vi "CalMic-Initialize Hardware.vi"(0 "Device":string, 5 "Params":T1, 11 "error in (no error)":errorcluster) -> (4 "task out":refnum<k21>, 6 "RPcoX out":refnum<k7>, 8 "npts":i32, 15 "error out":errorcluster)   [LabVIEW 2020]
uses:
  CalMic-Params.ctl
  epl-vi-lib/PXI DAQ VIs/TDT VIs/TDT-Signal Bank Action.ctl
  3100642b-de6f-4996-8a80-97bce8963f67.vi
  <vilib>/Comparison/Equal/Equal Functor/Equal Functor.lvclass
  <vilib>/DAQmx/create/channels.llb/DAQmx Create Channel (AI-Voltage-Basic).vi
  <vilib>/DAQmx/configure/timing.llb/DAQmx Timing (Sample Clock).vi
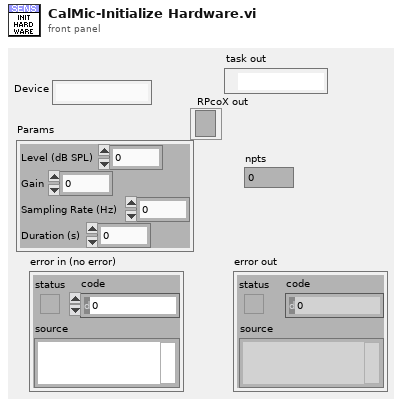
[diagram p1: front panel]
types:
  T1 = typedef "CalMic-Params.ctl" = cluster{"Level (dB SPL)":dbl, "Gain":dbl, "Sampling Rate (Hz)":dbl, "Duration (s)":dbl}
  T2 = typedef "TDT-Signal Bank Action.ctl" = enum16{"Init", "Write", "Read", "Rewrite", "Reset", "Recycle", "Ramp up", "Ramp down", "Zero"}
  T3 = typedef "TDT-Output source.ctl" = cluster{"Device":T4, "Num":i32}
  T4 = typedef "TDT-Device ID.ctl" = enum16{"None", "PA5", "RP2", "RL2", "RA16", "RV8", "RX5", "RX6", "RX7", "RX8", "RZ2", "RZ5", "RZ6"}
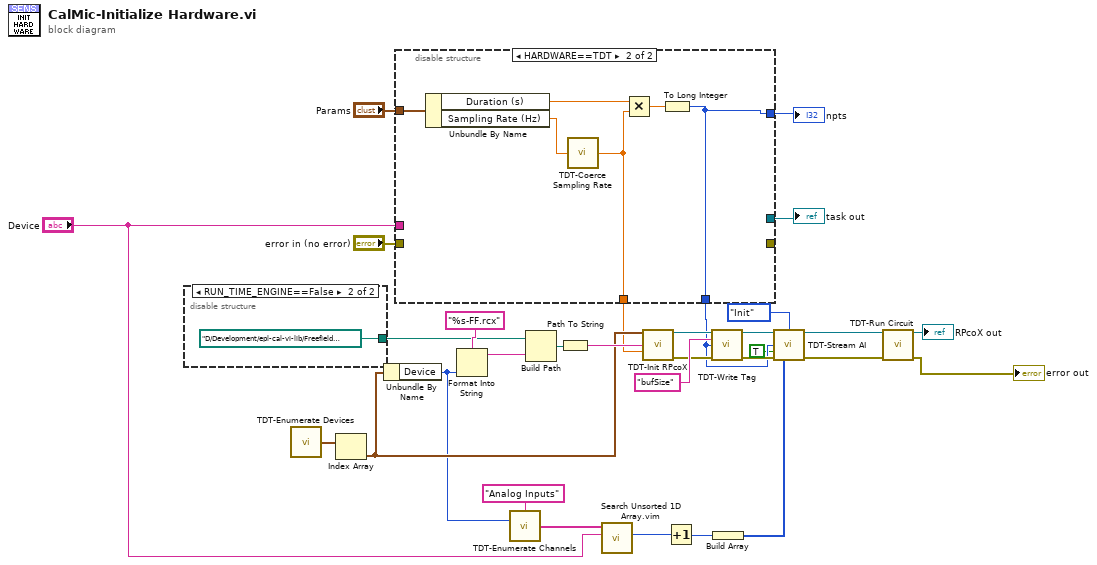
[diagram p0: block diagram]
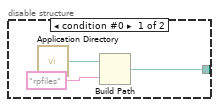
[diagram p2: hidden frame]
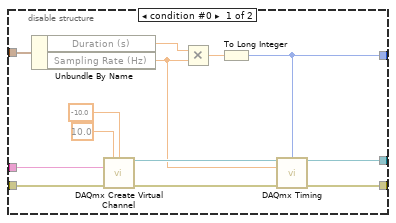
[diagram p3: hidden frame]
diagram:
  n1 = disable-structure shown="RUN_TIME_ENGINE==False" {
    disable-tunnel: [w33 path "D:/Development/epl-cal-vi-lib/Freefield Calibration VIs/rpfiles"] -> w23
    frame condition #0 {
      n2 = call <vilib>:"Application Directory.vi"() -> ("Application Directory"=w34:path)
      n3 = Build Path(base path=w34, name or relative path="rpfiles") -> (appended path=w33:path)
    }
    frame condition #1 (active) {
    }
  }
  n4 = call "TDT-Enumerate Devices.vi"() -> ("Devices"=w24:T3[])  [unwired: 14 in, 1 out]
  n5 = Index Array(array=w24) -> (element=w21:T3)  [unwired: 1 in]
  n6 = Unbundle By Name(w21) -> ("Device"=w15:T4)
  n7 = disable-structure shown="HARDWARE==TDT" {
    disable-tunnel: "Params" -> [w48 w52]
    disable-tunnel: "Device" -> [w47 _]
    disable-tunnel: "error in (no error)" -> [w44 _]
    disable-tunnel: [w38 w49] -> w29
    disable-tunnel: [w37 _] -> _
    disable-tunnel: [w36 _] -> w28
    disable-tunnel: [_ w50] -> w20
    disable-tunnel: [_ w49] -> w5
    frame condition #0 {
      n8 = Unbundle By Name(w48) -> ("Duration (s)"=w40:dbl, "Sampling Rate (Hz)"=w41:dbl)
      n9 = call-poly <vilib>:"DAQmx Create Virtual Channel.vi"("maximum value"=10.0, "minimum value"=-10.0, "physical channels"=w47, "error in"=w44) -> ("task out"=w43:refnum<k21>, "error out"=w42:errorcluster)  [unwired: 10 in]
      n10 = Multiply(x=w40, y=w41) -> (x*y=w39:dbl)
      n11 = To Long Integer(number=w39) -> (32bit integer=w38:i32)
      n12 = call-poly <vilib>:"DAQmx Timing.vi"("task/channels in"=w43, "samples per channel"=w38, "rate"=w41, "error in"=w42) -> ("task out"=w36:refnum<k21>, "error out"=w37:errorcluster)  [unwired: 10 in]
    }
    frame condition #1 (active) {
      n13 = Unbundle By Name(w52) -> ("Duration (s)"=w54:dbl, "Sampling Rate (Hz)"=w51:dbl)
      n14 = call "TDT-Coerce Sampling Rate.vi"("Fs (Hz)"=w51) -> ("Coerced"=w50:dbl)
      n15 = Multiply(x=w54, y=w50) -> (x*y=w53:dbl)
      n16 = To Long Integer(number=w53) -> (32bit integer=w49:i32)
    }
  }
  "npts" <- w29
  "task out" <- w28
  n17 = Format Into String(format string="%s-FF.rcx", w15) -> (resulting string=w26:string)  [unwired: 2 in, 1 out]
  n18 = call "TDT-Enumerate Channels.vi"("Type"="Analog Inputs", "IO Device"=w15) -> ("IO Channels"=w14:string[])  [unwired: 13 in]
  n19 = Build Path(base path=w23, name or relative path=w26) -> (appended path=w25:path)
  n20 = Path To String(path=w25) -> (string=w22:string)
  n21 = call "Search Unsorted 1D Array.vim"("element"="Device", "unsorted 1D array"=w14) -> ("index of element"=w8:i32)  [unwired: 9 in]
  n22 = call "TDT-Init RPcoX.vi"("Output"=w21, "RPfilename"=w22, "Sampling rate (Hz)"=w20) -> ("RPcoX"=w19:refnum<k7>, "error out"=w17:errorcluster)  [unwired: 11 in]
  n23 = Increment(x=w8) -> (x+1=w7:i32)
  n24 = call "TDT-Write Tag.vi"("RPcox"=w19, "Name"="bufSize", "Value"=w5, "error in"=w17) -> ("RPcox Out"=w12:refnum<k7>, "error out"=w11:errorcluster)  [unwired: 10 in]
  n25 = Build Array(w7) -> (w6:i32[])
  n26 = call "TDT-Stream AI.vi"("RPcox"=w12, "Action"=TDT-Signal_Bank_Action."Init", "Pts Per Read"=w5, "AI only"=TRUE, "error in (no error)"=w11, "AI Channels"=w6) -> ("RPcoX thru"=w10:refnum<k7>, "error out"=w4:errorcluster)  [unwired: 7 in, 1 out]
  n27 = call "TDT-Run Circuit.vi"("RPcoX"=w10, "error in (no error)"=w4) -> ("RPcoX out"=→"RPcoX out":refnum<k7>, "error out"=→"error out":errorcluster)  [unwired: 12 in]
